vi "Bdot JFT.vi"() -> ()   [LabVIEW 2020]
uses:
  <vilib>/addons/Time Frequency Analysis/_control.llb/TFA Configure Spectrogram Indicator (Predefined Color Table).vi
  <vilib>/addons/_Advanced Signal Processing/NI_AdvSigProcTFA.lvlib
  <vilib>/Analysis/NI_AALPro.lvlib
panel:
  out "Waveform Graph 2":waveform(dbl)(graph)
  out "Spectrogram":dbl[][](graph)
  in  "File Path":path
  out "Waveform Graph":waveform(dbl)(graph)
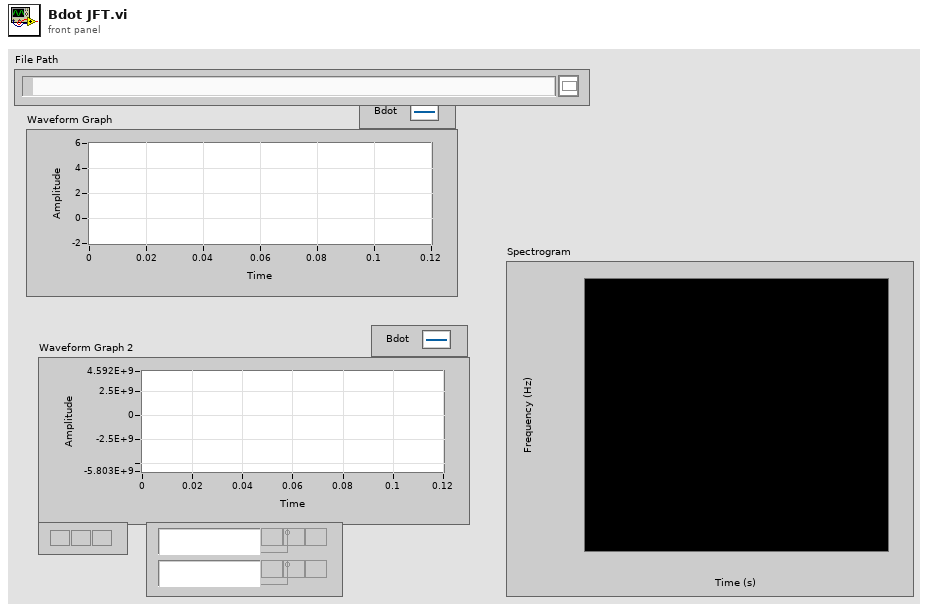
[diagram p1: front panel]
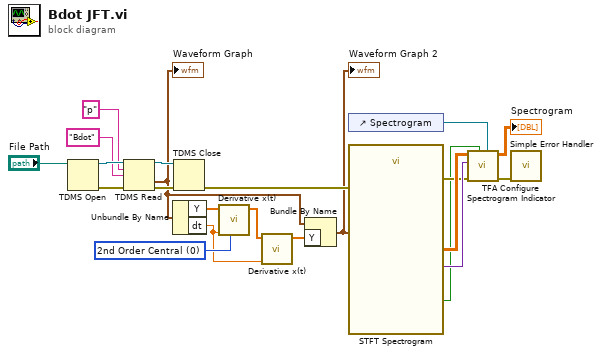
[diagram p0: block diagram]
diagram:
  w6 = u16 0 items=["2nd Order Central", "4th Order Central", "Forward", "Backward"] ("method")
  n1 = TDMS Open(11:"File Path") -> (0:w21:errorcluster, 3:w20:refnum<k34>)  [unwired: 6 in]
  n2 = TDMS Read(0:w20, 5:"p" ("group name in (Untitled)"), 7:"Bdot" ("group name in (Untitled)"), 11:w21) -> (4:w16:refnum<k34>, 10:w7:waveform(dbl), 15:w17:errorcluster)  [unwired: 4 in, 3 out]
  "Waveform Graph" <- w7
  n3 = Unbundle By Name(w7) -> ("Y"=w8:dbl[], "dt"=w2:dbl)
  n4 = TDMS Close(8:w17, 11:w16) -> (0:w15:errorcluster)  [unwired: 1 out]
  n5 = call <vilib>:"Derivative x(t).vi"("method"=w6, "dt"=w2, "X"=w8) -> ("dX/dt"=w4:dbl[])  [unwired: 7 in, 1 out]
  n6 = call <vilib>:"Derivative x(t).vi"("dt"=w2, "X"=w4) -> ("dX/dt"=w3:dbl[])  [unwired: 8 in, 1 out]
  n7 = Bundle By Name(cluster=w7, "Y"=w3) -> (w5:waveform(dbl))
  "Waveform Graph 2" <- w5
  n8 = control-ref of="Spectrogram"() -> (w12:refnum<vi>)
  n9 = call "STFT Spectrogram"("error in (no error)"=w15, "Signal"=w5) -> ("error out"=w10:errorcluster, "Scale Info"=w13:variant, "Spectrogram"=w14:dbl[][], "dB"=w1:bool)  [unwired: 5 in, 1 out]
  n10 = call-poly <vilib>:"TFA Configure Spectrogram Indicator.vi"("reference of TF spectrogram indicator"=w12, "dB on? (F)"=w1, "error in (no error)"=w10, "scale info"=w13, "spectrogram"=w14) -> ("error out"=w9:errorcluster, "TF spectrogram indicator"=→"Spectrogram":dbl[][])  [unwired: 2 in, 3 out]
  n11 = call <vilib>:"Simple Error Handler.vi"("error in (no error)"=w9) -> ()  [unwired: 4 in, 5 out]
